vi "read position of both axes.vi"(0 "GPIB # (in): def. 6":string, 3 "error in (no error)":errorcluster) -> (1 "fine axis (um)":ext[unit], 5 "fine axis (steps)":dbl, 6 "GPIB # (out)":string, 7 "coarse axis (um)":ext[unit], 8 "combined position (um)":ext[unit], 9 "coarse axis(steps)":dbl, 10 "error out":errorcluster)   [LabVIEW 2012]
uses:
  mc2mc4.llb/MC2/4 ReadPosition.VI
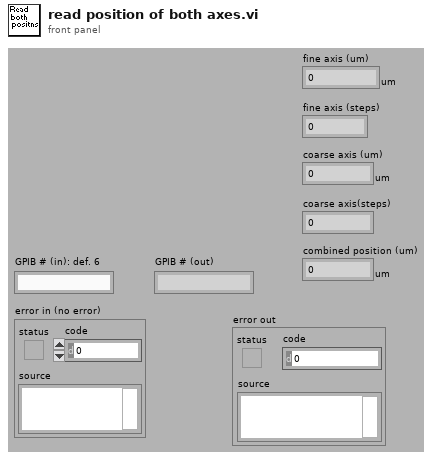
[diagram p1: front panel]
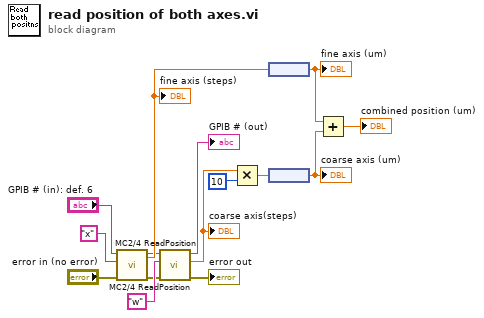
[diagram p0: block diagram]
diagram:
  n1 = call "MC2/4 ReadPosition.VI"("error in (no error)"="error in (no error)", "Axis"="x", "GPIB # (in): def. 6"="GPIB # (in): def. 6") -> ("error out"=w11:errorcluster, "Current Position"=w4:ext, "GPIB # (out)"=w2:string)  [unwired: 6 out]
  "fine axis (steps)" <- w4
  n2 = call "MC2/4 ReadPosition.VI"("error in (no error)"=w11, "Axis"="w", "GPIB # (in): def. 6"=w2) -> ("error out"=→"error out":errorcluster, "Current Position"=w5:ext, "GPIB # (out)"=→"GPIB # (out)":string)  [unwired: 6 out]
  "coarse axis(steps)" <- w5
  n3 = Multiply(x=w5, y=i8 10) -> (x*y=w10:ext)
  n4 = node(w4) -> (w8:ext[unit])
  "fine axis (um)" <- w8
  n5 = node(w10) -> (w7:ext[unit])
  "coarse axis (um)" <- w7
  n6 = Add(x=w8, y=w7) -> (x+y=→"combined position (um)":ext[unit])
